vi "Notes to index V2.vi"(0 "Notes In":string) -> (7 "Comments Out":string, 8 "output cluster":T1 {"Side Gate" items=["time", "Vsg", "T", "B", "X0", "Y0", "X1", "Y1", "X2", "Y2", "X3", "Y3", "X4", "Y4", "X5", "Y5", "B_rate", "R4t (e2/h)", "axis 1", "axis 2"]; "Current" items=["time", "Vsg", "T", "B", "X0", "Y0", "X1", "Y1", "X2", "Y2", "X3", "Y3", "X4", "Y4", "X5", "Y5", "B_rate", "R4t (e2/h)", "axis 1", "axis 2"]; "Voltage 1" items=["time", "Vsg", "T", "B", "X0", "Y0", "X1", "Y1", "X2", "Y2", "X3", "Y3", "X4", "Y4", "X5", "Y5", "B_rate", "R4t (e2/h)", "axis 1", "axis 2"]; "Voltage 2" items=["time", "Vsg", "T", "B", "X0", "Y0", "X1", "Y1", "X2", "Y2", "X3", "Y3", "X4", "Y4", "X5", "Y5", "B_rate", "R4t (e2/h)", "axis 1", "axis 2"]; "B Field" items=["time", "Vsg", "T", "B", "X0", "Y0", "X1", "Y1", "X2", "Y2", "X3", "Y3", "X4", "Y4", "X5", "Y5", "B_rate", "R4t (e2/h)", "axis 1", "axis 2"]})   [LabVIEW 2016]
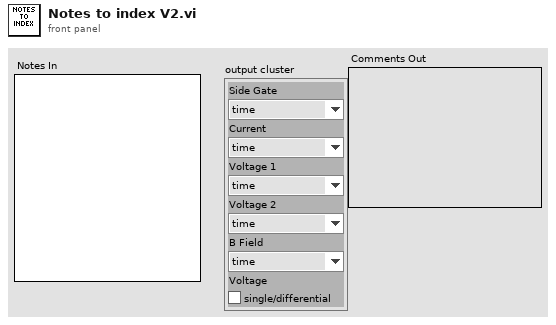
[diagram p1: front panel]
types:
  T1 = cluster{"Side Gate":i32, "Current":i32, "Voltage 1":i32, "Voltage 2":i32, "B Field":i32, "Voltage":bool}
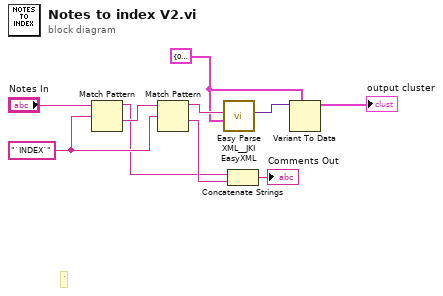
[diagram p0: block diagram]
diagram:
  w1 = T1 {"Side Gate"=0, "Current"=0, "Voltage 1"=0, "Voltage 2"=0, "B Field"=0, "Voltage"=FALSE} ("output cluster 2")
  w9 = "`INDEX`" ("regular expression")
  # "`"
  n1 = Match Pattern(string="Notes In", regular expression=w9) -> (before substring=w3:string, after substring=w10:string)  [unwired: 1 in, 2 out]
  n2 = Match Pattern(string=w10, regular expression=w9) -> (before substring=w7:string, after substring=w4:string)  [unwired: 1 in, 2 out]
  n3 = call <vilib>:"Easy Parse XML__JKI EasyXML.vi"("LabVIEW Data (Type)"=w1, "XML String"=w7) -> ("LabVIEW Data"=w6:variant)  [unwired: 8 in, 1 out]
  n4 = Concatenate Strings(w3, w4) -> (→"Comments Out":string)
  n5 = Variant To Data(type=w1, Variant=w6) -> (data=→"output cluster":T1)  [unwired: 1 in, 1 out]
